vi "MoveMemDeRefs.vi"() -> ()   [LabVIEW 2025]
uses:
  labview.exe
panel:
  out "addr 14":u64 format="%.0x"
  out "addr 13":u8[](array[numeric])
  out "addr 12":u64
  out "addr 11":u64
  out "addr 10":u64 format="%.0x"
  out "addr 9":u8[](array[numeric])
  out "addr 8":u8[](array[numeric])
  out "addr 7":u64 format="%.0x"
  out "addr 6":u8[](array[numeric])
  out "addr 5":u64 format="%.0x"
  out "addr 4":u8[](array[numeric])
  out "addr 3":u64 format="%.0x"
  out "addr 2":u8[](array[numeric])
  out "addr":u64 format="%.0x"
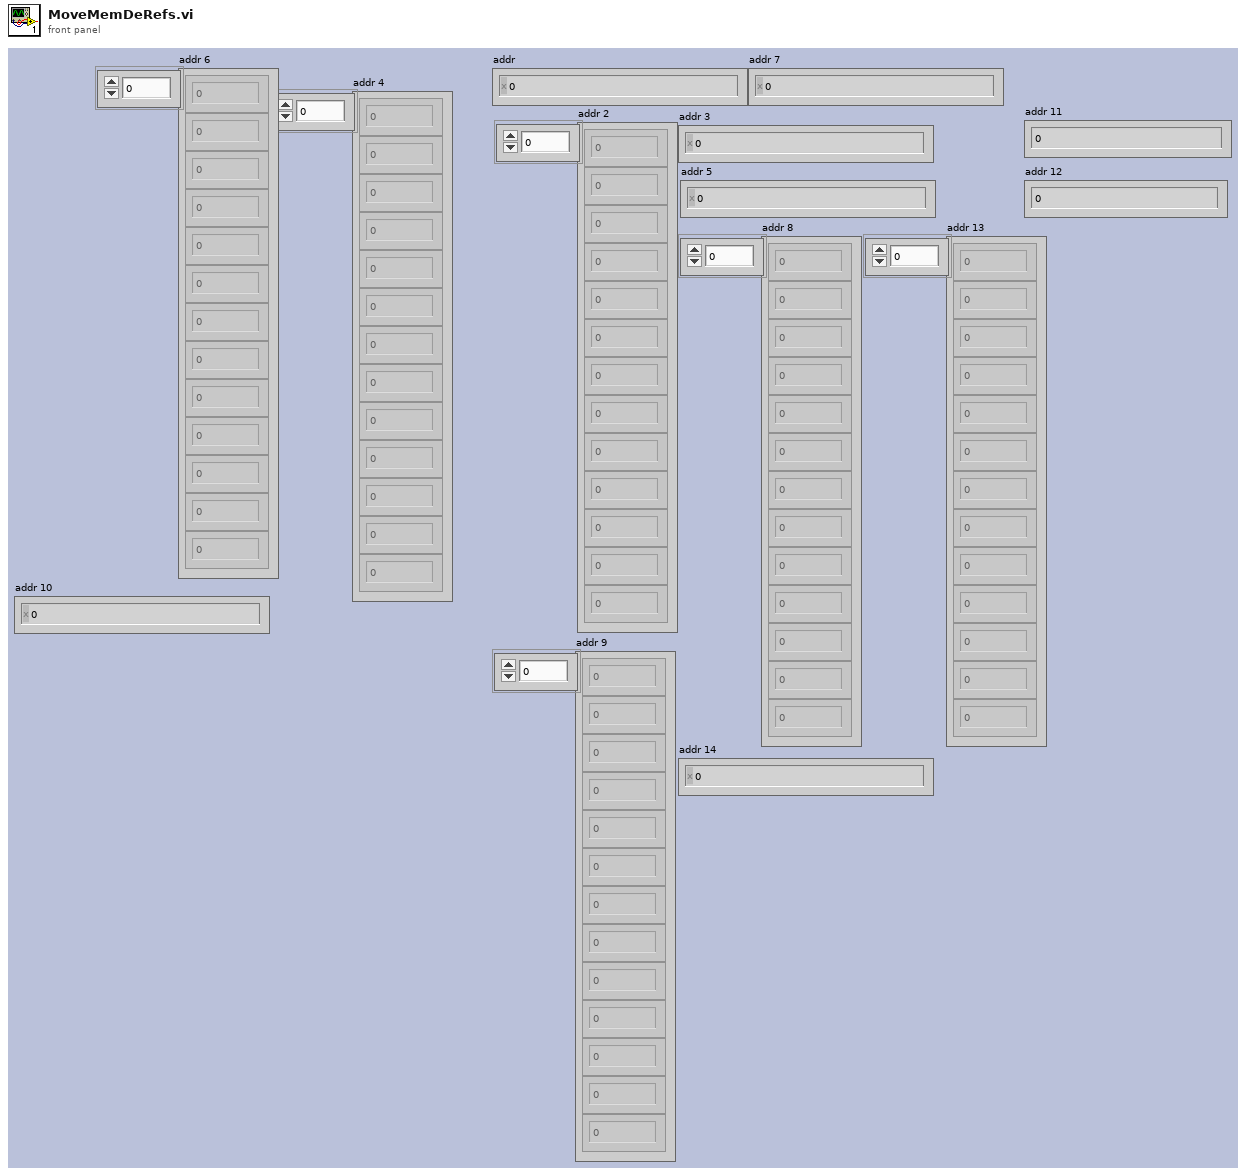
[diagram p1: front panel]
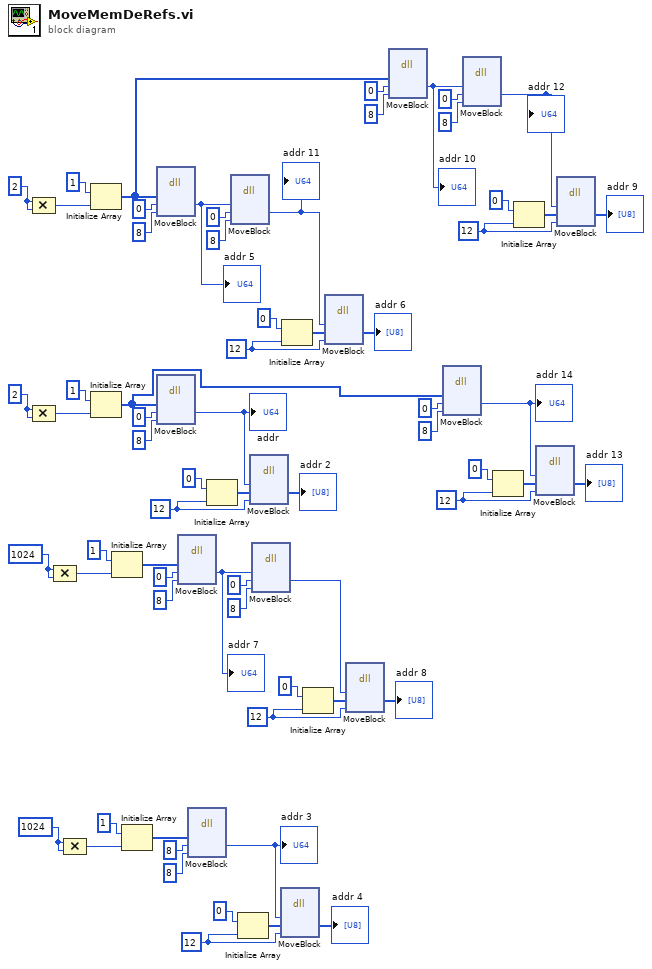
[diagram p0: block diagram]
diagram:
  w8 = 12 ("dimension size")
  w15 = 12 ("dimension size")
  w24 = 12 ("dimension size")
  w32 = 1024
  w38 = 12 ("dimension size")
  w45 = 2
  w47 = 12 ("dimension size")
  w56 = 1024
  w58 = 12 ("dimension size")
  w66 = 2
  n1 = Compound Arithmetic op=MULTIPLY(w45, w45) -> (w44:i32)
  n2 = Compound Arithmetic op=MULTIPLY(w66, w66) -> (w65:i32)
  n3 = Compound Arithmetic op=MULTIPLY(w32, w32) -> (w31:i32)
  n4 = Compound Arithmetic op=MULTIPLY(w56, w56) -> (w55:i32)
  n5 = Initialize Array(u8 1 ("element"), w44) -> (w9:u8[])
  n6 = Initialize Array(u8 1 ("element"), w65) -> (w1:u8[])
  n7 = Initialize Array(u8 1 ("element"), w31) -> (w30:u8[])
  n8 = Initialize Array(u8 1 ("element"), w55) -> (w54:u8[])
  n9 = dll-call lib="labview.exe" fn="MoveBlock"("arg1"=w9, "addr"=u64 0 ("arg3"), "arg3"=u64 8) -> ("addr"=w37:u64)  [unwired: 6 in, 2 out]
  "addr 5" <- w37
  n10 = dll-call lib="labview.exe" fn="MoveBlock"("arg1"=w1, "addr"=u64 0 ("arg3"), "arg3"=u64 8) -> ("addr"=w61:u64)  [unwired: 6 in, 2 out]
  "addr" <- w61
  n11 = dll-call lib="labview.exe" fn="MoveBlock"("arg1"=w30, "addr"=u64 0 ("arg3"), "arg3"=u64 8) -> ("addr"=w23:u64)  [unwired: 6 in, 2 out]
  "addr 7" <- w23
  n12 = dll-call lib="labview.exe" fn="MoveBlock"("arg1"=w54, "addr"=u64 8 ("arg3"), "arg3"=u64 8) -> ("addr"=w50:u64)  [unwired: 6 in, 2 out]
  "addr 3" <- w50
  n13 = Initialize Array(u8 0 ("element"), w58) -> (w60:u8[])
  n14 = dll-call lib="labview.exe" fn="MoveBlock"("arg1"=w37, "addr"=u64 0 ("arg3"), "arg3"=u64 8) -> ("addr"=w34:u64)  [unwired: 6 in, 2 out]
  "addr 11" <- w34
  n15 = Initialize Array(u8 0 ("element"), w47) -> (w49:u8[])
  n16 = dll-call lib="labview.exe" fn="MoveBlock"("arg1"=w61, "addr"=w60, "arg3"=w58) -> ("addr"=→"addr 2":u8[])  [unwired: 6 in, 2 out]
  n17 = dll-call lib="labview.exe" fn="MoveBlock"("arg1"=w23, "addr"=u64 0 ("arg3"), "arg3"=u64 8) -> ("addr"=w20:u64)  [unwired: 6 in, 2 out]
  n18 = dll-call lib="labview.exe" fn="MoveBlock"("arg1"=w50, "addr"=w49, "arg3"=w47) -> ("addr"=→"addr 4":u8[])  [unwired: 6 in, 2 out]
  n19 = Initialize Array(u8 0 ("element"), w38) -> (w40:u8[])
  n20 = Initialize Array(u8 0 ("element"), w24) -> (w26:u8[])
  n21 = dll-call lib="labview.exe" fn="MoveBlock"("arg1"=w34, "addr"=w40, "arg3"=w38) -> ("addr"=→"addr 6":u8[])  [unwired: 6 in, 2 out]
  n22 = dll-call lib="labview.exe" fn="MoveBlock"("arg1"=w20, "addr"=w26, "arg3"=w24) -> ("addr"=→"addr 8":u8[])  [unwired: 6 in, 2 out]
  n23 = dll-call lib="labview.exe" fn="MoveBlock"("arg1"=w9, "addr"=u64 0 ("arg3"), "arg3"=u64 8) -> ("addr"=w16:u64)  [unwired: 6 in, 2 out]
  "addr 10" <- w16
  n24 = dll-call lib="labview.exe" fn="MoveBlock"("arg1"=w1, "addr"=u64 0 ("arg3"), "arg3"=u64 8) -> ("addr"=w5:u64)  [unwired: 6 in, 2 out]
  "addr 14" <- w5
  n25 = dll-call lib="labview.exe" fn="MoveBlock"("arg1"=w16, "addr"=u64 0 ("arg3"), "arg3"=u64 8) -> ("addr"=w19:u64)  [unwired: 6 in, 2 out]
  "addr 12" <- w19
  n26 = Initialize Array(u8 0 ("element"), w8) -> (w6:u8[])
  n27 = Initialize Array(u8 0 ("element"), w15) -> (w13:u8[])
  n28 = dll-call lib="labview.exe" fn="MoveBlock"("arg1"=w5, "addr"=w6, "arg3"=w8) -> ("addr"=→"addr 13":u8[])  [unwired: 6 in, 2 out]
  n29 = dll-call lib="labview.exe" fn="MoveBlock"("arg1"=w19, "addr"=w13, "arg3"=w15) -> ("addr"=→"addr 9":u8[])  [unwired: 6 in, 2 out]
